vi "Custom Bias Sweep (pt by pt).vi"() -> ()   [LabVIEW 2021]
doc: "This example performs a custom bias sweep. You can create an array of Bias voltages and it will record the selected channels at each Bias voltage.\n\n- Nanonis Programming Interface -"
uses:
  Nanonis Prog Interface.lvlib
panel:
  in  "Settling time (ms)":u32=20 max=10000
  out "Steps done":i32=99
  out "XY Graph":cluster{dbl[], "Signals Values":sgl[]}(graph)={[1.0, 1.0101010101010102, 1.02020202020202, 1.0303030303030303, 1.0404040404040404, 1.0505050505050506, 1.0606060606060606, 1.0707070707070707, 1.0808080808080809, 1.0909090909090908, 1.101010101010101, 1.1111111111111112, 1.121212121212121, 1.1313131313131313, 1.1414141414141414, 1.1515151515151516, 1.1616161616161615, 1.1717171717171717, 1.1818181818181819, 1.191919191919192, 1.202020202020202, 1.2121212121212122, 1.2222222222222223, 1.2323232323232323, 1.2424242424242424, 1.2525252525252526, 1.2626262626262625, 1.2727272727272727, 1.2828282828282829, 1.2929292929292928, 1.303030303030303, 1.3131313131313131, 1.3232323232323233, 1.3333333333333335, 1.3434343434343434, 1.3535353535353536, 1.3636363636363638, 1.3737373737373737, 1.3838383838383839, 1.393939393939394, 1.404040404040404, 1.4141414141414141, 1.4242424242424243, 1.4343434343434343, 1.4444444444444444, 1.4545454545454546, 1.4646464646464648, 1.474747474747475, 1.4848484848484849, 1.494949494949495, 1.5050505050505052, 1.5151515151515151, 1.5252525252525253, 1.5353535353535355, 1.5454545454545454, 1.5555555555555556, 1.5656565656565657, 1.5757575757575757, 1.5858585858585859, 1.595959595959596, 1.606060606060606, 1.6161616161616164, 1.6262626262626263, 1.6363636363636365, 1.6464646464646466, 1.6565656565656566, 1.6666666666666667, 1.676767676767677, 1.6868686868686869, 1.696969696969697, 1.7070707070707072, 1.7171717171717171, 1.7272727272727273, 1.7373737373737375, 1.7474747474747474, 1.7575757575757578, 1.7676767676767677, 1.7777777777777777, 1.787878787878788, 1.797979797979798, 1.8080808080808082, 1.8181818181818183, 1.8282828282828283, 1.8383838383838385, 1.8484848484848486, 1.8585858585858586, 1.8686868686868687, 1.878787878787879, 1.8888888888888888, 1.8989898989898992, 1.9090909090909092, 1.9191919191919191, 1.9292929292929295, 1.9393939393939394, 1.9494949494949496, 1.9595959595959598, 1.9696969696969697, 1.97979797979798, 1.98989898989899, 2.0], "Signals Values"=[1.2042862e-11, 1.20325945e-11, 1.2290875e-11, 1.2495317e-11, 1.2677306e-11, 1.2855531e-11, 1.302402e-11, 1.3160834e-11, 1.3411918e-11, 1.3562116e-11, 1.3728125e-11, 1.3888775e-11, 1.4094991e-11, 1.4270381e-11, 1.44246325e-11, 1.4638239e-11, 1.4842029e-11, 1.50208e-11, 1.5230676e-11, 1.5388878e-11, 1.5604447e-11, 1.5804268e-11, 1.5968678e-11, 1.6173922e-11, 1.6409533e-11, 1.657843e-11, 1.6788949e-11, 1.6985654e-11, 1.7227811e-11, 1.7420291e-11, 1.7608344e-11, 1.779964e-11, 1.8047454e-11, 1.8277485e-11, 1.8483048e-11, 1.866429e-11, 1.8947986e-11, 1.9153156e-11, 1.9404277e-11, 1.9585729e-11, 1.987244e-11, 2.0078878e-11, 2.028474e-11, 2.0512626e-11, 2.0785694e-11, 2.1015545e-11, 2.1261973e-11, 2.1458902e-11, 2.1756399e-11, 2.1975638e-11, 2.216336e-11, 2.2471075e-11, 2.2769925e-11, 2.301386e-11, 2.3235882e-11, 2.3474202e-11, 2.3829088e-11, 2.4058176e-11, 2.4328914e-11, 2.4602738e-11, 2.4870394e-11, 2.5108346e-11, 2.5354347e-11, 2.5698147e-11, 2.60145e-11, 2.6240144e-11, 2.6606505e-11, 2.6829143e-11, 2.7220845e-11, 2.7433235e-11, 2.7800578e-11, 2.7986162e-11, 2.8410897e-11, 2.8689136e-11, 2.8967332e-11, 2.929488e-11, 2.9607598e-11, 2.989498e-11, 3.025324e-11, 3.0533638e-11, 3.094148e-11, 3.1261334e-11, 3.153527e-11, 3.193235e-11, 3.2308285e-11, 3.264748e-11, 3.2941153e-11, 3.3244723e-11, 3.3755554e-11, 3.4018545e-11, 3.439999e-11, 3.4753627e-11, 3.5155243e-11, 3.55296e-11, 3.5861404e-11, 3.6273363e-11, 3.6721175e-11, 3.7056858e-11, 3.743974e-11, 3.7750535e-11]}
  in  "Stop":bool
  in  "End (V)":dbl=2.0
  in  "Start (V)":dbl=1.0
  in  "N points":i32=100 min=2 max=10000
  # "Example program for the Nanonis SPM Control software programming interface\n\n - Custom Bias Sweep -"
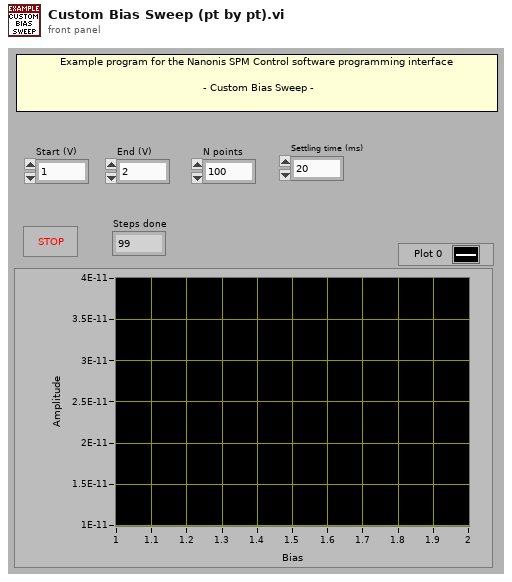
[diagram p1: front panel]
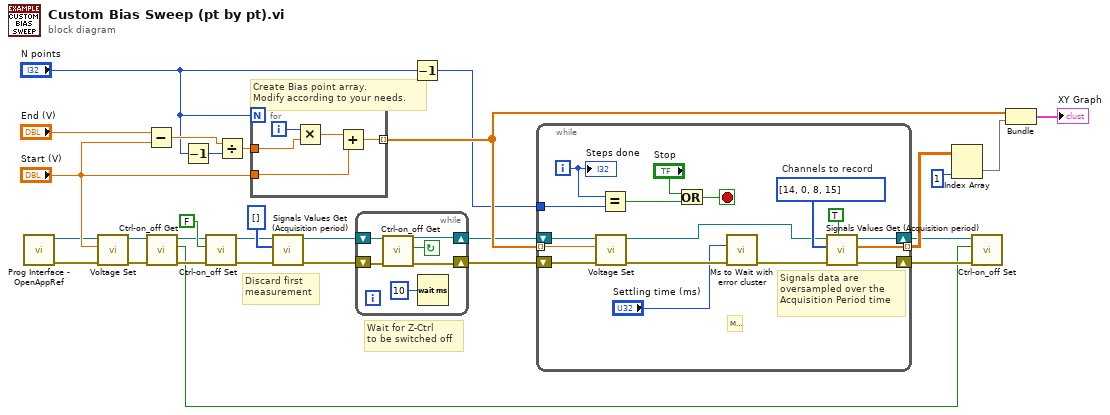
[diagram p0: block diagram]
diagram:
  # "Create Bias point array.\nModify according to your needs."
  # "Missing object. The object Loop Condition does not exist in the previous version."
  # "Wait for Z-Ctrl\nto be switched off"
  # "Discard first \nmeasurement"
  n1 = call <userlib>:"Prog Interface - OpenAppRef.vi"() -> ("Error out"=w20:errorcluster, "Application reference"=w8:refnum<vi>)  [unwired: 6 in]
  n2 = call <userlib>:"Voltage Set.vi"("Error in (no error)"=w20, "Bias (V)"="Start (V)", "Application ref in"=w8) -> ("Error out"=w16:errorcluster, "Application ref out"=w7:refnum<vi>)  [unwired: 7 in]
  n3 = Subtract(x="End (V)", y="Start (V)") -> (x-y=w28:dbl)
  n4 = call <userlib>:"Ctrl-on_off Get.vi"("error in (no error)"=w16, "Application ref in"=w7) -> ("error out"=w17:errorcluster, "Z-Controller on/off status"=w13:bool, "Application ref out"=w6:refnum<vi>)  [unwired: 7 in]
  n5 = Decrement(x="N points") -> (x-1=w26:i32)
  n6 = call <userlib>:"Ctrl-on_off Set.vi"("error in (no error)"=w17, "Z Controller ON/OFF"=FALSE, "Application ref in"=w6) -> ("error out"=w15:errorcluster, "Application ref out"=w4:refnum<vi>)  [unwired: 7 in]
  n7 = Divide(x=w28, y=w26) -> (x/y=w27:dbl)
  n8 = for {
    N: "N points" -> [_]
    tunnel: w27 -> [w33]
    tunnel: "Start (V)" -> [w31]
    tunnel: [w30] -> w22 mode=indexing
    i -> [w34]
    n9 = Multiply(x=w34, y=w33) -> (x*y=w32:dbl)
    n10 = Add(x=w32, y=w31) -> (x+y=w30:dbl)
  }
  n11 = call <userlib>:"Signals Values Get (Acquisition period).vi"("error in (no error)"=w15, "Signals indexes (0-127)"=i8[] [] ("Signals indexes (0-23)"), "Application ref in"=w4) -> ("error out"=w12:errorcluster, "Application ref out"=w3:refnum<vi>)  [unwired: 5 in, 1 out]
  n12 = while {
    shift-right: [w40] -> w11
    shift-left: w12 -> [w39]
    shift-right: [w35] -> w2
    shift-left: w3 -> [w36]
    stop <- w38 continue-if-true
    n13 = call <userlib>:"Ctrl-on_off Get.vi"("error in (no error)"=w39, "Application ref in"=w36) -> ("error out"=w40:errorcluster, "Z-Controller on/off status"=w38:bool, "Application ref out"=w35:refnum<vi>)  [unwired: 7 in]
    n14 = Wait (ms)(milliseconds to wait=u32 10) -> ()  [unwired: 1 out]
  }
  n15 = Decrement(x="N points") -> (x-1=w9:i32)
  n16 = while {
    tunnel: w22 -> [w57] mode=indexing
    tunnel: [w44] -> w25 mode=indexing
    shift-right: [w55] -> w14
    shift-left: w11 -> [w56]
    tunnel: w9 -> [w46]
    shift-right: [w43] -> w1
    shift-left: w2 -> [w45]
    i -> [w50]
    stop <- w47 stop-if-true
    w42 = i8[] [14, 0, 8, 15]  # Channels to record
    # "Signals data are \noversampled over the \nAcquisition Period time"
    n17 = call <userlib>:"Voltage Set.vi"("Error in (no error)"=w56, "Bias (V)"=w57, "Application ref in"=w45) -> ("Error out"=w54:errorcluster, "Application ref out"=w41:refnum<vi>)  [unwired: 7 in]
    n18 = Equal?(x=w50, y=w46) -> (x = y?=w49:bool)
    n19 = Or(x="Stop", y=w49) -> (x .or. y?=w47:bool)
    n20 = call "Ms to Wait with error cluster.vi"("error in (no error)"=w54, "milliseconds to wait"="Settling time (ms)") -> ("error out"=w53:errorcluster)  [unwired: 4 in, 1 out]
    n21 = call <userlib>:"Signals Values Get (Acquisition period).vi"("Wait for newest data (F=False)"=TRUE ("Wait for newest data (F)"), "error in (no error)"=w53, "Signals indexes (0-127)"=w42, "Application ref in"=w41) -> ("error out"=w55:errorcluster, "Signals Values"=w44:sgl[], "Application ref out"=w43:refnum<vi>)  [unwired: 4 in]
    "Steps done" <- w50
  }
  n22 = Index Array(array=w25, index (col)=1 ("disabled index (col)")) -> (element=w23:sgl[])  [unwired: 1 in]
  n23 = call <userlib>:"Ctrl-on_off Set.vi"("error in (no error)"=w14, "Z Controller ON/OFF"=w13, "Application ref in"=w1) -> ()  [unwired: 7 in, 2 out]
  n24 = Bundle(w22, "Signals Values"=w23) -> (→"XY Graph":cluster{dbl[], "Signals Values":sgl[]})  [unwired: 1 in]
